vi "XY Graph Find Threshold Location.vi"(8 "Error In":errorcluster, 9 "Threshold":dbl, 10 "Y Array":dbl[](array[numeric]), 11 "X Array":dbl[](array[numeric])) -> (0 "Error Out":errorcluster, 1 "Location Index":dbl, 3 "Threshold Location":dbl)   [LabVIEW 2021, in "XY Graph Add-Ons.lvlib"]
doc: "Finds the first element Yi in <B>Y Array</B> such that Yi >= <B>Threshold</B>.\n\nReturns the corresponding Xi as <B>Threshold Location</b> and, assuming a monotonously increasing <B>X Array</B>, the index of that element as <B>Location Index</b>.\n\nIf no value is found verifying this condition, the <B>Threshold Location</b> is NaN."
uses:
  <vilib>/Utility/error.llb/Error Cluster From Error Code.vi
  <vilib>/ErrorRing/Error Ring.xnode
  XY Graph Add-Ons.lvlib
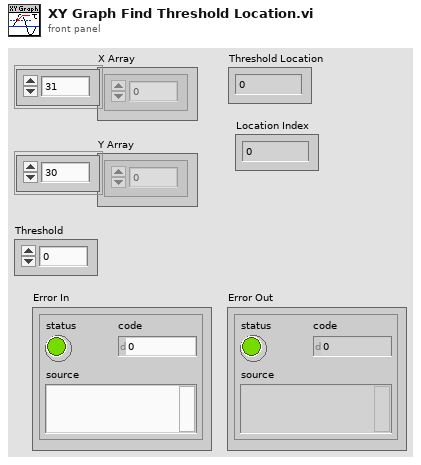
[diagram p1: front panel]
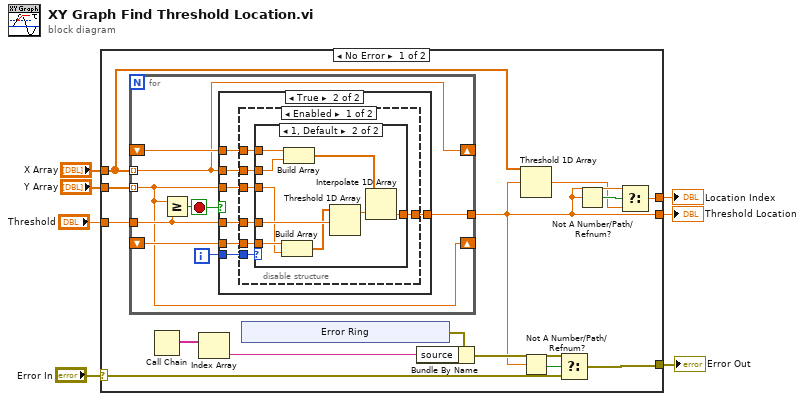
[diagram p0: block diagram]
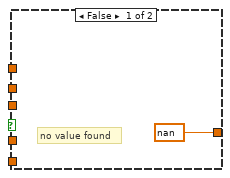
[diagram p2: hidden frame]
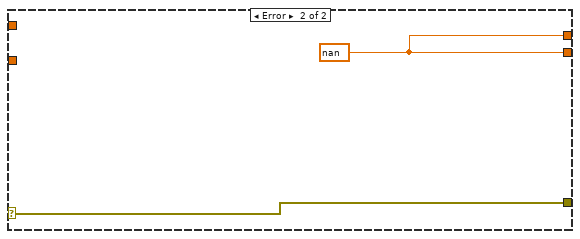
[diagram p5: hidden frame]
diagram:
  n1 = case shown="No Error" "Error In" {
    selector: "Error In" -> [w13 w60]
    tunnel: [w10 w61] -> w7
    tunnel: "Threshold" -> [w21 _]
    tunnel: "Y Array" -> [w20 _]
    tunnel: "X Array" -> [w19 _]
    tunnel: [w8 w61] -> w2
    tunnel: [w12 w60] -> w1
    frame No Error {
      n2 = for {
        tunnel: w19 -> [w29] mode=indexing
        tunnel: w20 -> [w31] mode=indexing
        tunnel: w21 -> [w33]
        shift-right: [w31] -> _
        shift-left: _ -> [w32]
        shift-right: [w29] -> _
        shift-left: _ -> [w30]
        tunnel: [w28] -> w10
        i -> [w26]
        stop <- w27 stop-if-true
        n3 = Greater Or Equal?(x=w31, y=w33) -> (x >= y?=w27:bool)
        n4 = case shown="True" w27 {
          tunnel: w33 -> [_ w41]
          tunnel: w32 -> [_ w40]
          tunnel: w31 -> [_ w39]
          tunnel: w30 -> [_ w38]
          tunnel: w29 -> [_ w37]
          tunnel: [nan w36] -> w28
          tunnel: w26 -> [_ w35]
          frame False {
            # "no value found"
          }
          frame True {
            n5 = disable-structure shown="Enabled" {
              disable-tunnel: w41 -> [w48 _]
              disable-tunnel: w40 -> [w47 _]
              disable-tunnel: w39 -> [w46 _]
              disable-tunnel: w38 -> [w45 _]
              disable-tunnel: w37 -> [w44 w59]
              disable-tunnel: [w43 w59] -> w36
              disable-tunnel: w35 -> [w42 _]
              frame Enabled {
                n6 = case shown="1, Default" w42 {
                  tunnel: w48 -> [_ w58]
                  tunnel: w47 -> [_ w56]
                  tunnel: w46 -> [_ w55]
                  tunnel: w45 -> [_ w54]
                  tunnel: w44 -> [w49 w53]
                  tunnel: [w49 w50] -> w43
                  frame 0 {
                  }
                  frame 1, Default {
                    n7 = Build Array(w56, w55) -> (w57:dbl[])
                    n8 = Build Array(w54, w53) -> (w52:dbl[])
                    n9 = Threshold 1D Array(2:w58, 3:w57) -> (0:w51:dbl)  [unwired: 1 in]
                    n10 = Interpolate 1D Array(1:w51, 2:w52) -> (0:w50:dbl)
                  }
                }
              }
              frame Disabled {
              }
            }
          }
        }
      }
      n11 = Call Chain() -> (call chain=w18:string[])
      n12 = Index Array(array=w18) -> (element=w17:string)  [unwired: 1 in]
      n13 = xnode "Error Ring"() -> ("error out"=w16:errorcluster)
      n14 = Bundle By Name(cluster=w16, "source"=w17) -> (w14:errorcluster)
      n15 = Threshold 1D Array(2:w10, 3:w19) -> (0:w9:dbl)  [unwired: 1 in]
      n16 = Not A Number/Path/Refnum?(number/path/refnum=w10) -> (NaN/Path/Refnum?=w15:bool)
      n17 = Select(t=w14, s=w15, f=w13) -> (s? t:f=w12:errorcluster)
      n18 = Not A Number/Path/Refnum?(number/path/refnum=w10) -> (NaN/Path/Refnum?=w11:bool)
      n19 = Select(t=w10, s=w11, f=w9) -> (s? t:f=w8:dbl)
    }
    frame Error {
      w61 = nan
    }
  }
  "Threshold Location" <- w7
  "Error Out" <- w1
  "Location Index" <- w2
